vi "SRV_Format Call Chain String.vi"(1 "Include This VI's Caller (T)":bool=TRUE) -> (8 "Formatted Call Chain String":string, 10 "Trimmed Call Chain":string[](array[string]))   [LabVIEW 2009]
doc: "Formats a call chain string; excluding this VI from the chain. If Include This VI's Caller is set to False, then it also excludes the caller of this VI from the chain.\n\n\nAuthor: Mike Schultz"
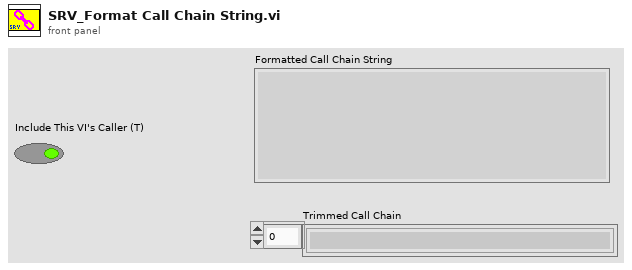
[diagram p1: front panel]
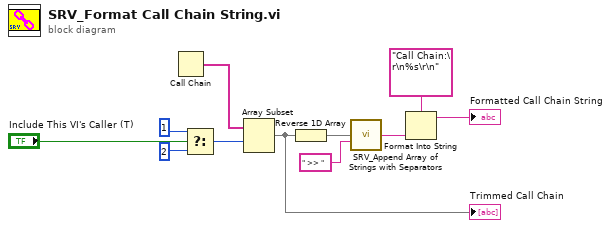
[diagram p0: block diagram]
diagram:
  n1 = Call Chain() -> (call chain=w5:string[])
  n2 = Select(t=1, s="Include This VI's Caller (T)", f=2) -> (s? t:f=w2:i32)
  n3 = Array Subset(array=w5, index=w2) -> (w9:string[])  [unwired: 1 in]
  "Trimmed Call Chain" <- w9
  n4 = Reverse 1D Array(array=w9) -> (reversed array=w10:string[])
  n5 = call "SRV_Append Array of Strings with Separators.vi"("Array of Strings to Append"=w10, "Element Separator(, )"=" >> ") -> ("String Out"=w7:string)  [unwired: 13 in]
  n6 = Format Into String(format string="Call Chain:\r\n%s\r\n", w7) -> (resulting string=→"Formatted Call Chain String":string)  [unwired: 2 in, 1 out]
